vi "Read FPGATarget.lvclass.vi"(8 "error in (no error)":errorcluster, 11 "FPGASession in":refnum<class "FPGASession.lvclass">) -> (0 "error out":errorcluster, 2 "FPGATarget.lvclass":refnum<class "FPGATarget.lvclass">, 3 "FPGASession out":refnum<class "FPGASession.lvclass">)   [LabVIEW 2013, in "FPGASession.lvclass"]
uses:
  FPGASession.lvclass
  FPGATargetClass/FPGATarget.lvclass
  FPGASession.lvclass/FPGASession.ctl
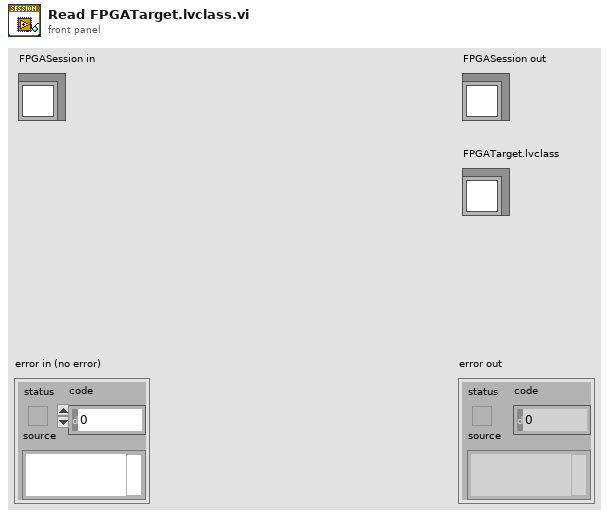
[diagram p1: front panel]
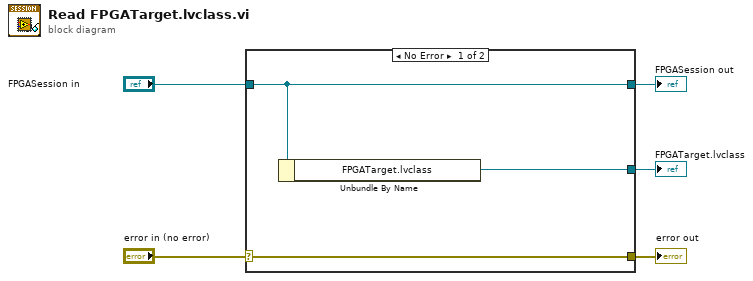
[diagram p0: block diagram]
diagram:
  n1 = case shown="No Error" "error in (no error)" {
    selector: "error in (no error)" -> [w8 w9]
    tunnel: [w8 w9] -> w4
    tunnel: [w7 w10] -> w2
    tunnel: "FPGASession in" -> [w7 w10]
    tunnel: [w6 _] -> w1
    frame No Error {
      n2 = Unbundle By Name(w7) -> ("FPGATarget.lvclass"=w6:refnum<class "FPGATarget.lvclass">)
    }
    frame Error {
    }
  }
  "error out" <- w4
  "FPGASession out" <- w2
  "FPGATarget.lvclass" <- w1
